vi "Scale Module (Main).vi"(7 "Name of Parent Panel":string="Main.vi", 9 "New Center Coords":T1={"Horizontal"=470, "Vertical"=200}, 10 "Config":variant, 11 "Main UI Message Queue":refnum<queue>) -> ()   [LabVIEW 2018, in "Scale Module.lvlib"]
doc: "This Continuous Measurement sample project is based on the Queued Message Handler template.\n\nThe Event Handling Loop generates messages based on user interface actions.\n\nThe Message Handling Loop processes messages generated by the Event Handling Loop, or by other messages. There are also Acquisition and Logging message handling loop subVIs, and a chart updating loop."
uses:
  Scale Module.lvlib
  support/Message Queue/Message Cluster.ctl
  <vilib>/Utility/miscctls.llb/LVPoint32TypeDef.ctl
  controls/UI State.ctl
  Feed Module/Controls/Scale Module Config Cluster.ctl
  Feed Module/Controls/Scale Module Settings Cluster.ctl
  Mettler Toledo/Controls/Settings Cluster.ctl
  Feed Module/Controls/Scale Module State Cluster.ctl
  Feed Module/Controls/Scale Module Display.ctl
  support/Message Queue/Enqueue Message (Single).vi
  <vilib>/Utility/error.llb/Error Cluster From Error Code.vi
  <vilib>/ErrorRing/Error Ring.xnode
  support/User Event - Stop/User Event - Stop.lvlib
  support/Message Queue/Message Queue.lvlib
  support/Support Library.lvlib
  Measure Instrument/Scale Module Engine.lvlib
  Mettler Toledo/Mettler Toledo.lvlib
  Scale Settings Dialog.vi
  support/Command Log VIs/Command Logging.lvlib
panel:
  in  "Settings Button":bool
  out "ScanCode":i16
  out "g":dbl format="%#_5f"
  out "Log File path":path
  out "Status":string
  in  "Exit":bool
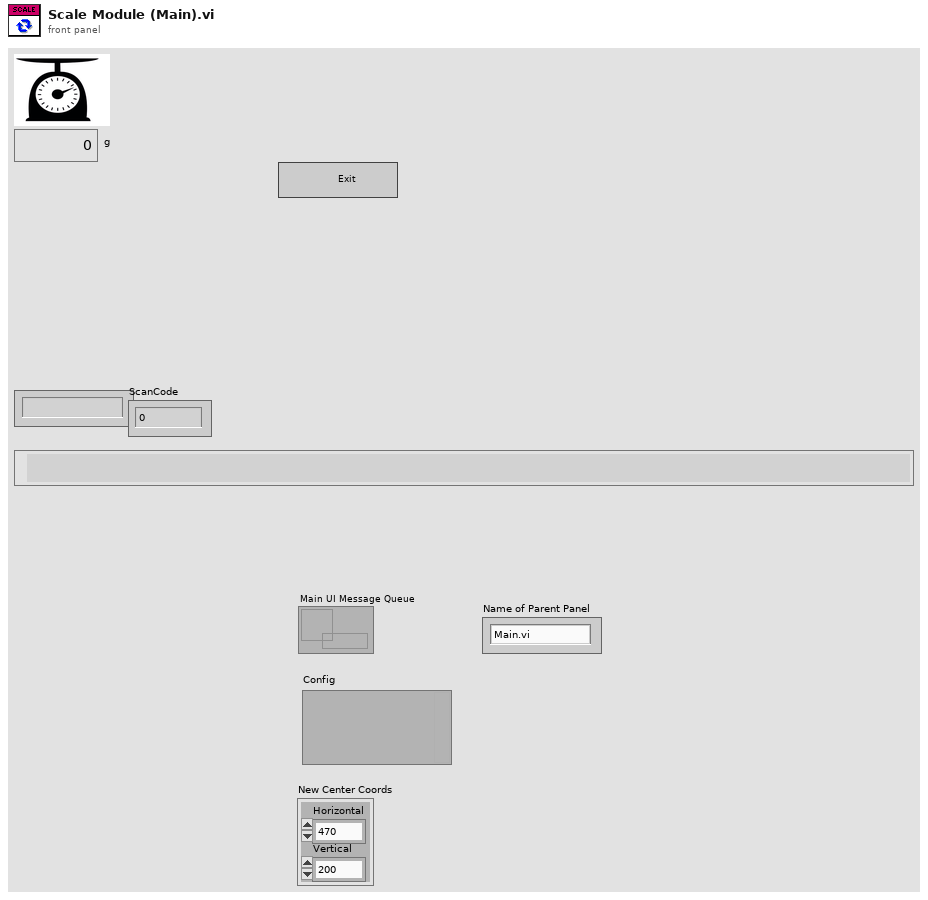
[diagram p1: front panel]
types:
  T1 = typedef "LVPoint32TypeDef.ctl" = cluster{"Horizontal":i32, "Vertical":i32}
  T2 = typedef "Scale Module.lvlib/Scale Module State Cluster.ctl" = cluster{"Scale Module Config":T3}
  T3 = typedef "Scale Module.lvlib/Scale Module Config Cluster.ctl" = cluster{"GUID":string, "Drop Coords":T1, "Process Name":string, "Queue Name":string, "Settings":T4, "Load Count":i32}
  T4 = typedef "Scale Module.lvlib/Scale Module Settings Cluster.ctl" = cluster{"Cycle Period":dbl, "Mettler":T5, "Scale Type":string}
  T5 = typedef "Mettler Toledo.lvlib/Settings Cluster.ctl" = cluster{"VISA resource name":refnum<visa-resource-name>, "Simulated?":bool}
  T6 = typedef "UI State.ctl" = enum16{"Idle", "Acquiring and Logging", "Waiting for Exit", "Waiting for Exit (Acq Stopped)", "Waiting for Exit (Log Stopped)", "Waiting for Stop", "Waiting for Stop (Acq Stopped)", "Waiting for Stop (Log Stopped)"}
  T7 = typedef "Scale Module.lvlib/Scale Message Queues.ctl" = cluster{"Scale UI":refnum<queue>, "Scale Engine":refnum<queue>, "Scale Display":refnum<queue>}
  T8 = typedef "Scale Module.lvlib/Scale Module Display.ctl" = cluster{"Scale Value":dbl, "Cycle Period":dbl}
  T9 = cluster{"Shift":bool, "Ctrl":bool, "Alt":bool, "Cmd":bool, "Opt":bool}
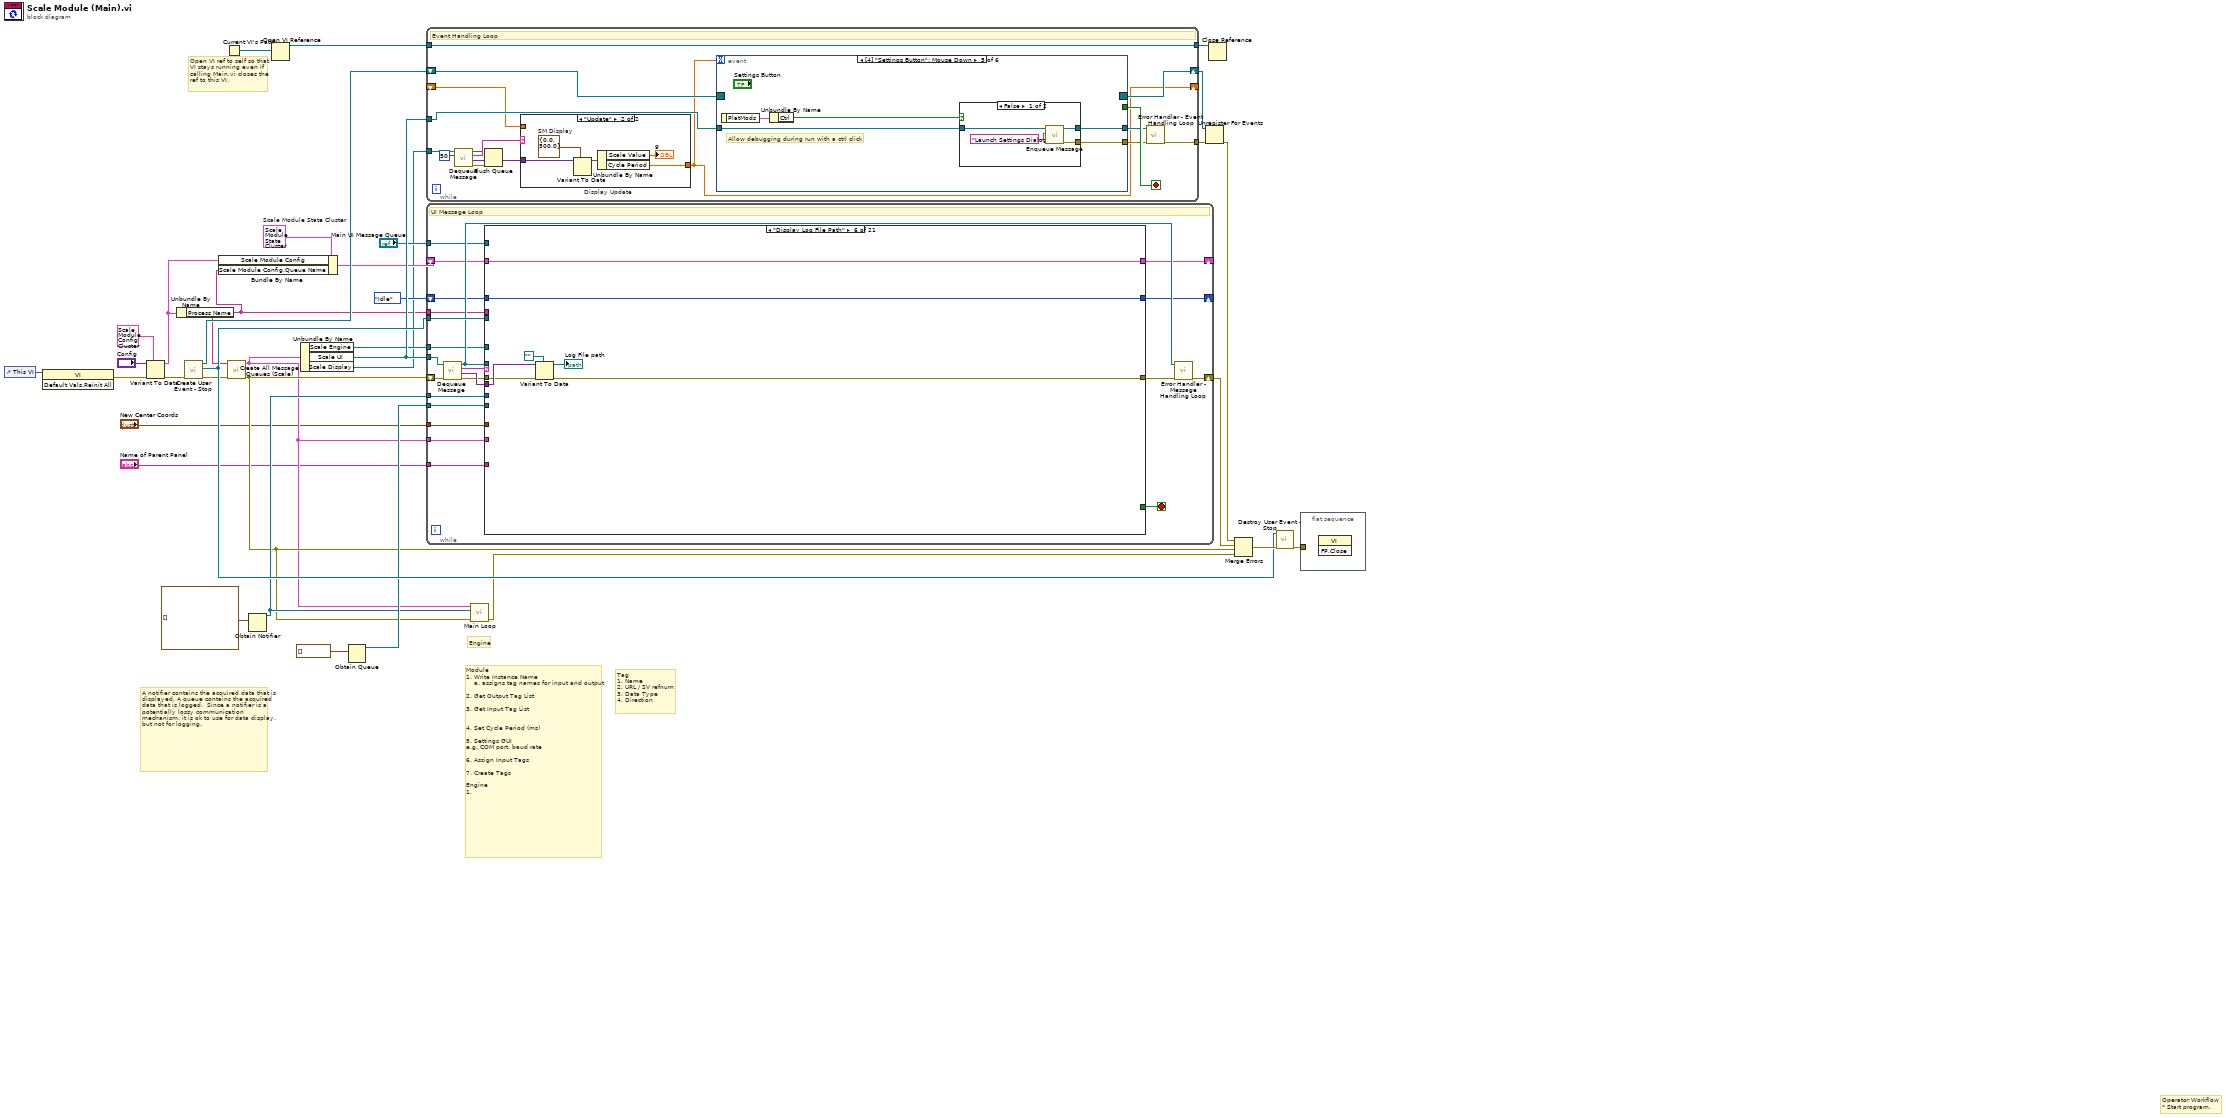
[diagram p0: block diagram]
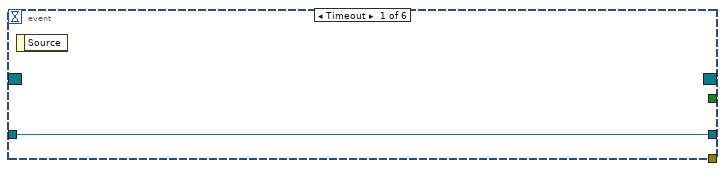
[diagram p3: hidden frame]
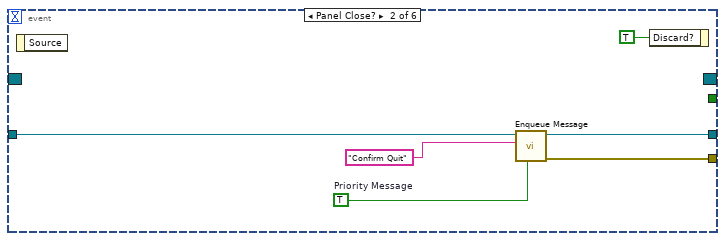
[diagram p4: hidden frame]
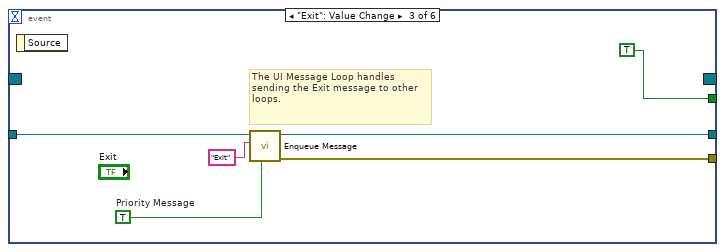
[diagram p5: hidden frame]
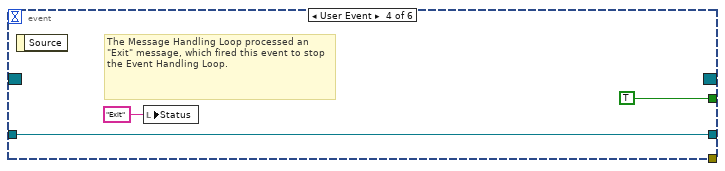
[diagram p6: hidden frame]
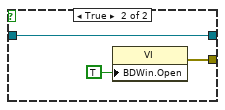
[diagram p7: hidden frame]
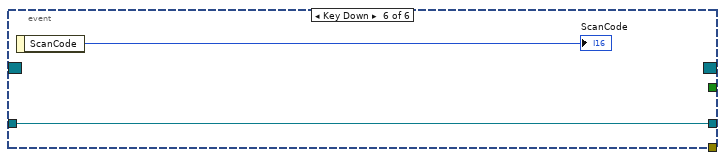
[diagram p8: hidden frame]
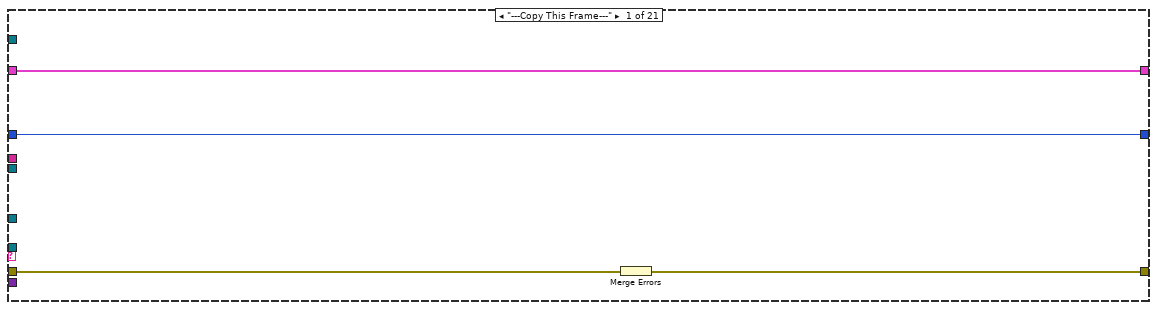
[diagram p9: hidden frame]
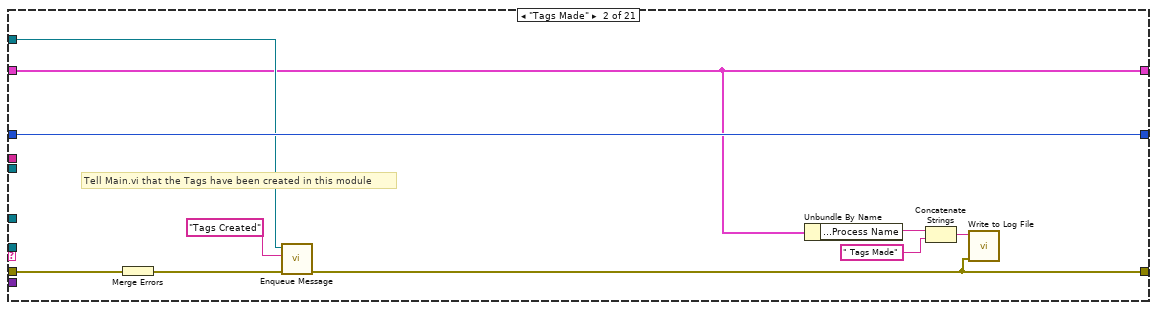
[diagram p10: hidden frame]
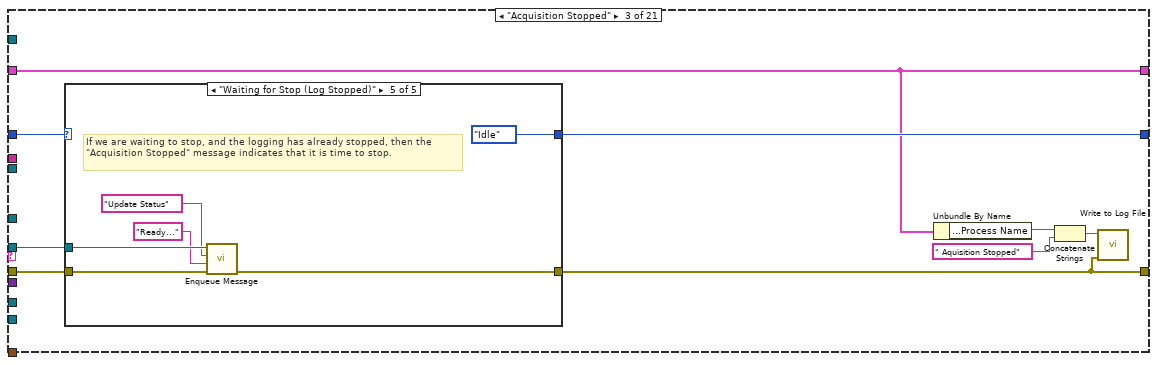
[diagram p11: hidden frame]
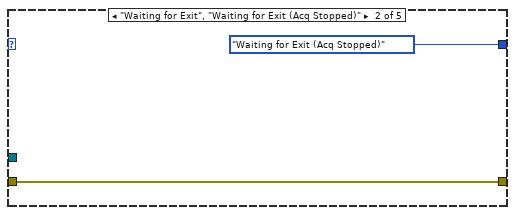
[diagram p13: hidden frame]
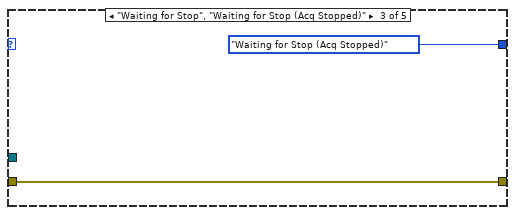
[diagram p14: hidden frame]
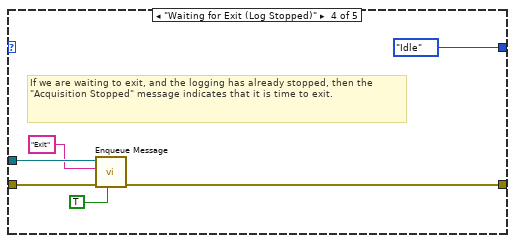
[diagram p15: hidden frame]
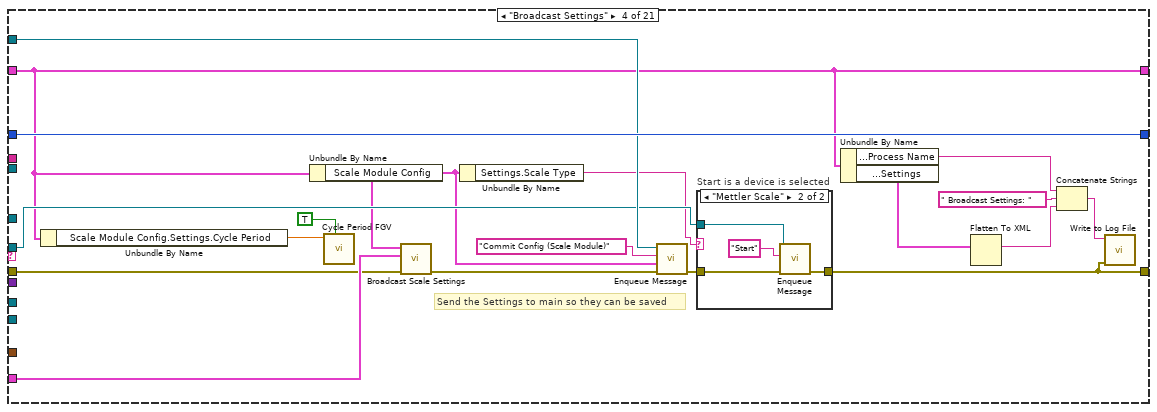
[diagram p16: hidden frame]
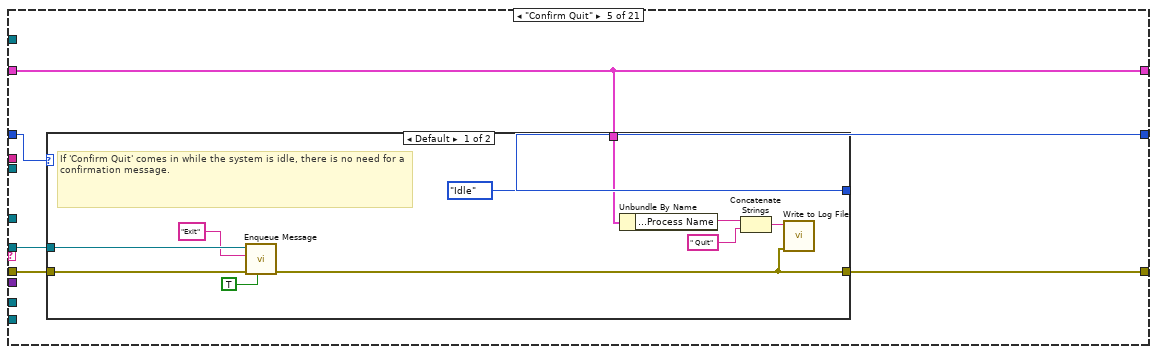
[diagram p18: hidden frame]
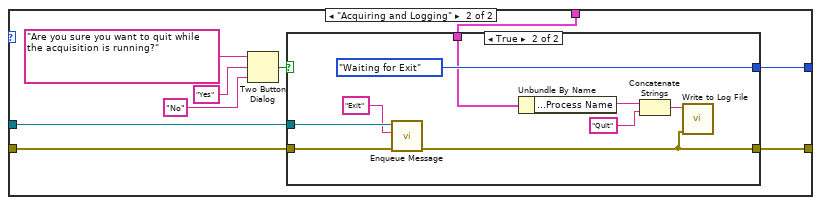
[diagram p19: hidden frame]
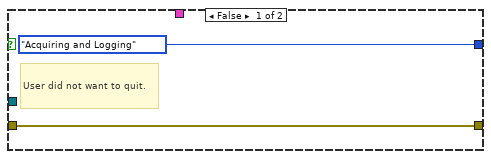
[diagram p20: hidden frame]
diagram:
  w13 = T2 {"Scale Module Config"={"GUID"="PID1-Mettler Toledo Scale 1", "Drop Coords"={"Horizontal"=0, "Vertical"=0}, "Process Name"="PID1-Setpoint", "Queue Name"="", "Settings"={"Cycle Period"=500.0, "Mettler"={"VISA resource name"="", "Simulated?"=FALSE}, "Scale Type"=""}, "Load Count"=0}}  # Scale Module State Cluster
  # "Open VI ref to self so that\nVI stays running even if\ncalling Main.vi closes the\nref to this VI."
  # "Engine"
  # "Operator Workflow\n* Start program."
  # "Module \n1. Write Instance Name\n    a. assigns tag names for input and output\n\n2. Get Output Tag List\n\n3. Get Input Tag List\n\n\n4. Set Cycle Period (ms)\n\n5. Settings GUI\ne.g. COM port, baud rate\n\n6. Assign Input Tags\n\n7. Create Tags\n\nEngine\n1."
  # "Tag\n1. Name\n2. URL / SV refnum\n3. Data Type\n4. Direction"
  # "A notifier contains the acquired data that is displayed. A queue contains the acquired data that is logged.  Since a notifier is a potentially lossy communication mechanism, it is ok to use for data display, but not for logging."
  n1 = control-ref of="This VI"() -> (w10:refnum<vi>)
  n2 = invoke class="VI" method="Default Vals.Reinit All"(reference=w10) -> (error out=w2:errorcluster)  [unwired: 2 in, 2 out]
  n3 = Variant To Data(error in=w2, type=T3 {"GUID"="", "Drop Coords"={"Horizontal"=0, "Vertical"=0}, "Process Name"="", "Queue Name"="", "Settings"={"Cycle Period"=500.0, "Mettler"={"VISA resource name"="", "Simulated?"=FALSE}, "Scale Type"=""}, "Load Count"=0} ("Feed Module Config"), Variant="Config") -> (data=w11:T3, error out=w16:errorcluster)
  n4 = Unbundle By Name(w11) -> ("Process Name"=w1:string)
  n5 = call "Create User Event - Stop.vi"("error in (no error)"=w16) -> ("error out"=w8:errorcluster, "User Event - Stop"=w31:refnum<user-event>, "Stop Event Registration Refnum"=w32:refnum<event-registration>)  [unwired: 8 in]
  n6 = Bundle By Name(cluster=w13, "Scale Module Config"=w11, "Scale Module Config.Queue Name"=w1) -> (w17:T2)
  n7 = Current VI's Path() -> (path=w18:path)
  n8 = call "Create All Message Queues (Scale).vi"("error in (no error)"=w8, "Process Name"=w1) -> ("error out"=w7:errorcluster, "Message Queues"=w6:T7)  [unwired: 8 in]
  n9 = Obtain Notifier(notification data type=waveform(dbl)[] []) -> (notifier out=w21:refnum<notifier>)  [unwired: 3 in, 2 out]
  n10 = Open VI Reference(vi path=w18) -> (vi reference=w19:refnum<vi>)  [unwired: 5 in, 1 out]
  n11 = Unbundle By Name(w6) -> ("Scale Engine"=w24:refnum<queue>, "Scale UI"=w28:refnum<queue>, "Scale Display"=w12:refnum<queue>)
  n12 = Obtain Queue(element data type=waveform(dbl)[] []) -> (queue out=w23:refnum<queue>)  [unwired: 4 in, 2 out]
  n13 = while {
    tunnel: w28 -> [w52]
    tunnel: w31 -> [w56]
    shift-right: [w48] -> w35
    shift-left: w7 -> [w55]
    shift-right: [w39] -> _
    shift-left: w17 -> [w41]
    tunnel: w21 -> [w51]
    tunnel: w23 -> [w50]
    shift-right: [w45] -> _
    shift-left: UI_State."Idle" ("UI State") -> [w46]
    tunnel: w24 -> [w44]
    tunnel: w6 -> [w43]
    tunnel: "Main UI Message Queue" -> [w40]
    tunnel: w1 -> [w38]
    tunnel: "New Center Coords" -> [w37]
    tunnel: "Name of Parent Panel" -> [w36]
    stop <- w57 stop-if-true
    # "UI Message Loop"
    n14 = call "Dequeue Message.vi"("error in (no error)"=w55, "Message Queue"=w52) -> ("error out"=w42:errorcluster, "Message Data"=w53:variant, "Message"=w54:string, "dup Message Queue"=w47:refnum<queue>)  [unwired: 6 in]
    n15 = case "Message Cases" shown="\"Display Log File Path\"" w54 {
      selector: w54 -> [_ _ _ _ _ _ _ _ _ _ _ _ _ _ _ _ _ _ _ _ w393]
      tunnel: w47 -> [_ _ w77 w109 w127 _ w177 w191 w213 _ w252 w269 w286 w309 w317 w335 _ _ w382 _ _]
      tunnel: w42 -> [w61 w71 w78 w113 w126 w161 w172 w195 w212 w238 w248 w267 w287 w310 w316 w334 w341 w358 w377 w391 _]
      tunnel: [w60 w62 w73 w102 w125 w162 w167 w182 w197 w238 w240 w260 w282 w308 w315 w330 w346 w353 w369 w392 w395] -> w49
      tunnel: [_ _ _ _ _ _ _ _ TRUE _ _ _ _ _ _ _ _ _ _ _ _] -> w57
      tunnel: w53 -> [_ _ _ _ _ w164 _ w194 w202 _ _ _ _ _ _ _ _ _ _ w390 _]
      tunnel: w56 -> [_ _ _ _ _ _ _ _ w223 _ _ _ _ _ _ _ _ _ _ _ _]
      tunnel: w41 -> [w58 w63 w72 w101 w123 w159 w166 w181 w196 w235 w239 w271 w281 w314 w321 w329 w339 w352 w368 w385 w394]
      tunnel: w51 -> [_ _ _ _ _ _ _ _ w221 _ _ _ _ _ _ _ _ _ _ _ _]
      tunnel: w50 -> [_ _ _ _ _ _ _ _ w217 _ _ _ _ _ _ _ _ _ _ _ _]
      tunnel: w46 -> [w59 w70 w80 w117 w128 w160 w173 w186 w210 _ _ w275 w289 w313 w320 _ _ _ w378 w386 w399]
      tunnel: [w59 w70 w79 w117 w124 w160 w174 w186 w209 UI_State."Idle" ("UI State") UI_State."Idle" ("UI State") w275 w288 w313 w320 UI_State."Acquiring and Logging" ("UI State") UI_State."Acquiring and Logging" ("UI State") UI_State."Acquiring and Logging" ("UI State") w379 w386 w399] -> w45
      tunnel: w44 -> [_ _ _ _ _ _ _ _ w216 _ _ _ _ _ _ _ w344 w361 w376 _ _]
      tunnel: w43 -> [_ _ _ w116 _ _ _ _ _ _ _ _ _ _ _ _ _ _ _ _ _]
      tunnel: w40 -> [_ w67 _ w110 _ _ _ _ w201 _ _ w272 _ _ _ _ _ _ _ _ _]
      tunnel: [w58 w63 w72 w101 w123 w159 w166 w181 w196 w235 w239 w259 w281 w314 w321 w329 w339 w352 w368 w385 w394] -> w39
      tunnel: w38 -> [_ _ _ _ _ _ _ _ _ _ w246 _ _ _ _ _ _ _ _ _ _]
      tunnel: w37 -> [_ _ _ _ _ _ _ _ _ _ w245 _ _ _ _ _ _ _ _ _ _]
      tunnel: w36 -> [_ _ _ _ _ _ _ _ _ _ w244 _ _ _ _ _ _ _ _ _ _]
      frame "---Copy This Frame---" {
        # "Duplicate this frame when creating new messages.  Change this comment in the duplicated frame to describe this message."
        n16 = Merge Errors(w61) -> (w60:errorcluster)
      }
      frame "Tags Made" {
        # "Tell Main.vi that the Tags have been created in this module"
        # "Duplicate this frame when creating new messages.  Change this comment in the duplicated frame to describe this message."
        n17 = Merge Errors(w71) -> (w68:errorcluster)
        n18 = call-poly "Enqueue Message.vi"("error in (no error)"=w68, "Message"="Tags Created", "Message Queue"=w67) -> ("error out"=w62:errorcluster)  [unwired: 7 in, 1 out]
        n19 = Unbundle By Name(w63) -> ("Scale Module Config.Process Name"=w66:string)
        n20 = Concatenate Strings(w66, " Tags Made" ("text")) -> (w64:string)
        n21 = call "Write to Log File.vi"("error in"=w62, "text"=w64) -> ()  [unwired: 9 in, 1 out]
      }
      frame "Acquisition Stopped" {
        # "Logic for determining what action to take when the acquisition has stopped."
        n22 = case shown="\"Waiting for Stop (Log Stopped)\"" w80 {
          selector: w80 -> [w82 _ _ _ _]
          tunnel: [w82 UI_State."Waiting for Exit (Acq Stopped)" ("UI State") UI_State."Waiting for Stop (Acq Stopped)" ("UI State") UI_State."Idle" ("UI State") UI_State."Idle" ("UI State")] -> w79
          tunnel: w78 -> [w81 w83 w85 w91 w97]
          tunnel: [w81 w83 w85 w90 w96] -> w73
          tunnel: w77 -> [_ _ _ w89 w95]
          frame Default {
          }
          frame "Waiting for Exit", "Waiting for Exit (Acq Stopped)" {
          }
          frame "Waiting for Stop", "Waiting for Stop (Acq Stopped)" {
          }
          frame "Waiting for Exit (Log Stopped)" {
            # "If we are waiting to exit, and the logging has already stopped, then the \"Acquisition Stopped\" message indicates that it is time to exit."
            n23 = call-poly "Enqueue Message.vi"("Priority Message? (F)"=TRUE, "error in (no error)"=w91, "Message"="Exit", "Message Queue"=w89) -> ("error out"=w90:errorcluster)  [unwired: 6 in, 1 out]
          }
          frame "Waiting for Stop (Log Stopped)" {
            # "If we are waiting to stop, and the logging has already stopped, then the \"Acquisition Stopped\" message indicates that it is time to stop."
            n24 = call-poly "Enqueue Message.vi"("error in (no error)"=w97, "Message Data"="Ready..." ("Message"), "Message"="Update Status", "Message Queue"=w95) -> ("error out"=w96:errorcluster)  [unwired: 6 in, 1 out]
          }
        }
        n25 = Unbundle By Name(w72) -> ("Scale Module Config.Process Name"=w76:string)
        n26 = Concatenate Strings(w76, " Aquisition Stopped" ("text")) -> (w74:string)
        n27 = call "Write to Log File.vi"("error in"=w73, "text"=w74) -> ()  [unwired: 9 in, 1 out]
      }
      frame "Broadcast Settings" {
        # "Send the Settings to main so they can be saved"
        # "Send the 'Update Settings' message to the Logging and Acquisition message loops."
        n28 = Unbundle By Name(w101) -> ("Scale Module Config.Settings.Cycle Period"=w114:dbl)
        n29 = Unbundle By Name(w101) -> ("Scale Module Config"=w106:T3)
        n30 = call "Cycle Period FGV.vi"("Write"=TRUE, "Cycle Period In (ms)"=w114) -> ()  [unwired: 8 in, 2 out]
        n31 = call "Broadcast Scale Settings.vi"("error in (no error)"=w113, "Message Queues"=w116, "Scale Module Config"=w106) -> ("error out"=w111:errorcluster)  [unwired: 8 in]
        n32 = Unbundle By Name(w106) -> ("Settings.Scale Type"=w107:string)
        n33 = call-poly "Enqueue Message.vi"("error in (no error)"=w111, "Message Data"=w106, "Message"="Commit Config (Scale Module)", "Message Queue"=w110) -> ("error out"=w108:errorcluster)  [unwired: 6 in, 1 out]
        n34 = case "Start is a device is selected" shown="\"Mettler Scale\"" w107 {
          tunnel: w109 -> [_ w121]
          tunnel: w108 -> [w118 w120]
          tunnel: [w118 w119] -> w102
          frame "False", Default {
          }
          frame "Mettler Scale" {
            n35 = call-poly "Enqueue Message.vi"("error in (no error)"=w120, "Message"="Start", "Message Queue"=w121) -> ("error out"=w119:errorcluster)  [unwired: 7 in, 1 out]
          }
        }
        n36 = Unbundle By Name(w101) -> ("Scale Module Config.Process Name"=w105:string, "Scale Module Config.Settings"=w100:T4)
        n37 = Flatten To XML(anything=w100) -> (xml string=w99:string)
        n38 = Concatenate Strings(w105, " Broadcast Settings: " ("text"), w99) -> (w103:string)
        n39 = call "Write to Log File.vi"("error in"=w102, "text"=w103) -> ()  [unwired: 9 in, 1 out]
      }
      frame "Confirm Quit" {
        # "Confirm Quit - Message that can confirm whether or not the user wants to exit the application."
        n40 = case shown="Default" w128 {
          tunnel: w127 -> [w137 w144]
          tunnel: w126 -> [w136 w142]
          tunnel: [w130 w141] -> w125
          tunnel: [UI_State."Idle" ("UI State") w140] -> w124
          tunnel: w123 -> [w129 w139]
          frame Default {
            # "If 'Confirm Quit' comes in while the system is idle, there is no need for a confirmation message."
            n41 = call-poly "Enqueue Message.vi"("Priority Message? (F)"=TRUE, "error in (no error)"=w136, "Message"="Exit", "Message Queue"=w137) -> ("error out"=w130:errorcluster)  [unwired: 6 in, 1 out]
            n42 = Unbundle By Name(w129) -> ("Scale Module Config.Process Name"=w133:string)
            n43 = Concatenate Strings(w133, " Quit" ("text")) -> (w131:string)
            n44 = call "Write to Log File.vi"("error in"=w130, "text"=w131) -> ()  [unwired: 9 in, 1 out]
          }
          frame "Acquiring and Logging" {
            n45 = Two Button Dialog(message="Are you sure you want to quit while the acquisition is running?" ("Confirm Quit Message"), 1:"No" ("No"), 2:"Yes" ("Yes")) -> (T button?=w143:bool)
            n46 = case shown="True" w143 {
              tunnel: w144 -> [_ w158]
              tunnel: w142 -> [w148 w157]
              tunnel: [w148 w151] -> w141
              tunnel: [UI_State."Acquiring and Logging" ("UI State") UI_State."Waiting for Exit" ("UI State")] -> w140
              tunnel: w139 -> [_ w150]
              frame False {
                # "User did not want to quit."
              }
              frame True {
                n47 = call-poly "Enqueue Message.vi"("error in (no error)"=w157, "Message"="Exit", "Message Queue"=w158) -> ("error out"=w151:errorcluster)  [unwired: 7 in, 1 out]
                n48 = Unbundle By Name(w150) -> ("Scale Module Config.Process Name"=w154:string)
                n49 = Concatenate Strings(w154, "Quit" ("text")) -> (w152:string)
                n50 = call "Write to Log File.vi"("error in"=w151, "text"=w152) -> ()  [unwired: 9 in, 1 out]
              }
            }
          }
        }
      }
      frame "Display Log File Path" {
        n51 = Variant To Data(error in=w161, type=path "", Variant=w164) -> (data=→"Log File path":path, error out=w162:errorcluster)
      }
      frame "E-Stop" {
        # "E-Stop has no effect on the scale"
        # "Message Acquisition and Logging loops to stop"
        # "Stop the pumps."
        n52 = call-poly "Enqueue Message.vi"("error in (no error)"=w172, "Message Data"="Ready..." ("Ready..."), "Message"="Update Status", "Message Queue"=w177) -> ("error out"=w171:errorcluster)  [unwired: 6 in, 1 out]
        n53 = case shown="\"Waiting for Exit\"" w173 {
          selector: w173 -> [_ w179]
          tunnel: [UI_State."Waiting for Stop" ("UI State") w179] -> w174
          frame Default {
          }
          frame "Waiting for Exit" {
          }
        }
        n54 = Merge Errors(w171) -> (w167:errorcluster)
        n55 = Unbundle By Name(w166) -> ("Scale Module Config.Process Name"=w170:string)
        n56 = Concatenate Strings(w170, " E-STOP" ("text")) -> (w168:string)
        n57 = call "Write to Log File.vi"("error in"=w167, "text"=w168) -> ()  [unwired: 9 in, 1 out]
      }
      frame "Error" {
        # "Error - Check the error message data and respond accordingly. This message is sent by the \"Error Handler\" VIs at the end of each loop in this application."
        n58 = Variant To Data(error in=w195, type=errorcluster {"status"=FALSE, "code"=0, "source"=""} ("error out"), Variant=w194) -> (data=w192:errorcluster, error out=w188:errorcluster)
        n59 = call <vilib>:"General Error Handler.vi"("error in (no error)"=w192) -> ("message"=w180:string)  [unwired: 10 in, 4 out]
        n60 = call-poly "Enqueue Message.vi"("Priority Message? (F)"=TRUE, "Message"="Exit", "Message Queue"=w191) -> ("error out"=w187:errorcluster)  [unwired: 7 in, 1 out]
        n61 = Merge Errors(w187, w188) -> (w182:errorcluster)
        n62 = Unbundle By Name(w181) -> ("Scale Module Config.Process Name"=w185:string)
        n63 = Concatenate Strings(w185, " Error: " ("text"), w180) -> (w183:string)
        n64 = call "Write to Log File.vi"("error in"=w182, "text"=w183) -> ()  [unwired: 9 in, 1 out]
      }
      frame "Exit" {
        w205 = TRUE  # Delete Module?
        # "Don't check the error outs. The acquisition and logging queues may have already been released."
        # "Close references owned by the Main VI."
        # "Stop the VI"
        # "Exit - Fire the User Event to stop the Event Handling Loop.  Also send Exit messages to the Acquisition and Logging loops."
        n65 = call "Fire User Event - Stop.vi"("User Event - Stop"=w223) -> ("error out"=w222:errorcluster)  [unwired: 10 in]
        n66 = Build Array(w216) -> (w215:refnum<queue>[])
        n67 = for {
          tunnel: w215 -> [w232] mode=indexing
          n68 = call-poly "Enqueue Message.vi"("Message"="Stop", "Message Queue"=w232) -> ("dup Message Queue"=w233:refnum<queue>)  [unwired: 8 in, 1 out]
          n69 = call-poly "Enqueue Message.vi"("Message"="Exit", "Message Queue"=w233) -> ()  [unwired: 8 in, 2 out]
        }
        n70 = Variant To Data(type=w205, Variant=w202) -> (data=w204:bool, error out=w206:errorcluster)  [unwired: 1 in]
        n71 = call-poly "Enqueue Message.vi"("error in (no error)"=w212, "Message Data"="Ready..." ("Ready..."), "Message"="Update Status", "Message Queue"=w213) -> ("error out"=w211:errorcluster, "dup Message Queue"=w208:refnum<queue>)  [unwired: 6 in]
        n72 = Select(t=w205, s=w206, f=w204) -> (s? t:f=w203:bool)
        n73 = case "Don't enqueue Delete Module if opening campaign because it\nwill already have been deleted and new config loaded and we create\na race condition." shown="True" w203 {
          tunnel: w201 -> [_ w227]
          tunnel: w196 -> [_ w226]
          frame False {
          }
          frame True {
            n74 = Unbundle By Name(w226) -> ("Scale Module Config.GUID"=w225:string)
            n75 = call-poly "Enqueue Message.vi"("Message Data"=w225, "Message"="Delete Module", "Message Queue"=w227) -> ()  [unwired: 7 in, 2 out]
          }
        }
        n76 = Release Queue(queue=w208, error in (no error)=w211) -> (error out=w220:errorcluster)  [unwired: 1 in, 2 out]
        n77 = Release Notifier(notifier=w221, error in (no error)=w220) -> (error out=w219:errorcluster)  [unwired: 1 in, 2 out]
        n78 = Release Queue(queue=w217, error in (no error)=w219) -> (error out=w218:errorcluster)  [unwired: 1 in, 2 out]
        n79 = Merge Errors(w222, w218) -> (w197:errorcluster)
        n80 = case shown="Default" w210 {
          selector: w210 -> [_ w230]
          tunnel: [UI_State."Waiting for Stop" ("UI State") w230] -> w209
          frame Default {
          }
          frame "Waiting for Exit" {
          }
        }
        n81 = Unbundle By Name(w196) -> ("Scale Module Config.Process Name"=w200:string)
        n82 = Concatenate Strings(w200, " Exit" ("text")) -> (w198:string)
        n83 = call "Write to Log File.vi"("error in"=w197, "text"=w198) -> ()  [unwired: 9 in, 1 out]
      }
      frame "Init UI Refs" {
        # "Init UI Refs - Store control references for UI controls.  Also enable/disable controls appropriately."
        n84 = property class="VI"("Front Panel.Closeable"=TRUE ("Front Panel Window:Closeable")) -> ()  [unwired: 2 in, 2 out]
      }
      frame "Initialize" {
        # "Initialize - Get configuration settings, then message the UI to initialize, and broadcast the settings to the other message loops."
        n85 = call-poly "Enqueue Message.vi"("error in (no error)"=w248, "Message"="Init UI Refs", "Message Queue"=w252) -> ("error out"=w250:errorcluster, "dup Message Queue"=w251:refnum<queue>)  [unwired: 7 in]
        n86 = property class="VI" props=["FP.State"]() -> (reference out=w247:refnum<vi>)  [unwired: 2 in, 2 out]
        n87 = call "Make Child and Move.vi"("Process Name"=w246, "Name of Parent Panel"=w244, "New Center Coords"=w245, "VI in"=w247) -> ()  [unwired: 8 in]
        n88 = call-poly "Enqueue Message.vi"("error in (no error)"=w250, "Message"="Broadcast Settings", "Message Queue"=w251) -> ("error out"=w258:errorcluster, "dup Message Queue"=w257:refnum<queue>)  [unwired: 7 in]
        n89 = call-poly "Enqueue Message.vi"("error in (no error)"=w258, "Message Data"="Ready..." ("Ready..."), "Message"="Update Status", "Message Queue"=w257) -> ("error out"=w240:errorcluster)  [unwired: 6 in, 1 out]
        n90 = Unbundle By Name(w239) -> ("Scale Module Config.Process Name"=w243:string)
        n91 = Concatenate Strings(w243, " Initialize" ("text")) -> (w241:string)
        n92 = call "Write to Log File.vi"("error in"=w240, "text"=w241) -> ()  [unwired: 9 in, 1 out]
      }
      frame "Launch Settings Dialog" {
        # "Launch the Settings Dialog when the user clicks the 'Settings' button."
        n93 = Unbundle By Name(w271) -> ("Scale Module Config"=w270:T3)
        n94 = Unbundle By Name(w270) -> ("Load Count"=w273:i32)
        n95 = Increment(x=w273) -> (x+1=w274:i32)
        n96 = Bundle By Name(cluster=w270, "Load Count"=w274) -> (w268:T3)
        n97 = call-by-ref "?"("error in (no error)"=w267, "Scale Module Config In"=w268) -> ("error out"=w266:errorcluster, "Cancelled?"=w264:bool, "Scale Module Config Out"=w265:T3)  [unwired: 8 in, 3 out]
        n98 = case shown="False" w264 {
          tunnel: w266 -> [w277 w280]
          tunnel: [w276 w280] -> w260
          tunnel: w272 -> [_ _]
          tunnel: w269 -> [w279 _]
          tunnel: w265 -> [_ _]
          frame False {
            n99 = call-poly "Enqueue Message.vi"("error in (no error)"=w277, "Message"="Broadcast Settings", "Message Queue"=w279) -> ("error out"=w276:errorcluster)  [unwired: 7 in, 1 out]
          }
          frame True {
          }
        }
        n100 = Bundle By Name(cluster=w271, "Scale Module Config"=w265) -> (w259:T2)
        n101 = Unbundle By Name(w259) -> ("Scale Module Config.Process Name"=w263:string)
        n102 = Concatenate Strings(w263, " Setting Dialog Launched" ("text")) -> (w261:string)
        n103 = call "Write to Log File.vi"("error in"=w260, "text"=w261) -> ()  [unwired: 9 in, 1 out]
      }
      frame "Logging Stopped" {
        # "Logic for determining what action to take when the logging has stopped."
        n104 = case shown="\"Waiting for Exit (Acq Stopped)\"" w289 {
          selector: w289 -> [w291 _ _ _ _]
          tunnel: [w291 UI_State."Waiting for Exit (Log Stopped)" ("UI State") UI_State."Waiting for Stop (Log Stopped)" ("UI State") UI_State."Idle" ("UI State") UI_State."Idle" ("UI State")] -> w288
          tunnel: w287 -> [w290 w292 w294 w300 w306]
          tunnel: [w290 w292 w294 w299 w305] -> w282
          tunnel: w286 -> [_ _ _ w298 w304]
          frame Default {
          }
          frame "Waiting for Exit", "Waiting for Exit (Log Stopped)" {
          }
          frame "Waiting for Stop", "Waiting for Stop (Log Stopped)" {
          }
          frame "Waiting for Exit (Acq Stopped)" {
            # "If we are waiting to exit, and the acquisition has already stopped, then the \"Logging Stopped\" message indicates that it is time to exit."
            n105 = call-poly "Enqueue Message.vi"("Priority Message? (F)"=TRUE, "error in (no error)"=w300, "Message"="Exit", "Message Queue"=w298) -> ("error out"=w299:errorcluster)  [unwired: 6 in, 1 out]
          }
          frame "Waiting for Stop (Acq Stopped)" {
            # "If we are waiting to stop, and the acquisition has already stopped, then the \"Logging Stopped\" message indicates that it is time to stop."
            n106 = call-poly "Enqueue Message.vi"("error in (no error)"=w306, "Message Data"="Ready..." ("Message"), "Message"="Update Status", "Message Queue"=w304) -> ("error out"=w305:errorcluster)  [unwired: 6 in, 1 out]
          }
        }
        n107 = Unbundle By Name(w281) -> ("Scale Module Config.Process Name"=w285:string)
        n108 = Concatenate Strings(w285, " Logging Stopped" ("text")) -> (w283:string)
        n109 = call "Write to Log File.vi"("error in"=w282, "text"=w283) -> ()  [unwired: 9 in, 1 out]
      }
      frame "Send to Sequencer" {
        n110 = local read "g"() -> (w311:dbl)
        n111 = call-poly "Enqueue Message.vi"("error in (no error)"=w310, "Message Data"=w311, "Message"="Sent to Sequence", "Message Queue"=w309) -> ("error out"=w308:errorcluster)  [unwired: 6 in, 1 out]
      }
      frame "Sent to Sequence" {
        n112 = local read "g"() -> (w318:dbl)
        n113 = flat-sequence {
          tunnel: w316 -> [w326]
          tunnel: w317 -> [w324]
          tunnel: [w325] -> w319
          tunnel: w318 -> [w322]
          tunnel: [w328] -> w315
          tunnel: w319 -> [w328]
          frame #0 {
            n114 = call-poly "Enqueue Message.vi"("error in (no error)"=w326, "Message Data"=w322, "Message"="Sent to Sequence", "Message Queue"=w324) -> ("error out"=w325:errorcluster)  [unwired: 6 in, 1 out]
          }
          frame #1 {
            n115 = Wait (ms)(milliseconds to wait=u32 50) -> ()  [unwired: 1 out]
          }
        }
      }
      frame "Start" {
        # "Message Acquisition and Logging loops to start"
        # "Start - Enable/Disable buttons appropriately for an acquisition that has started, and update status display."
        n116 = call-poly "Enqueue Message.vi"("error in (no error)"=w334, "Message"="Start Loops", "Message Queue"=w335) -> ("error out"=w336:errorcluster)  [unwired: 7 in, 1 out]
        n117 = Merge Errors(w336) -> (w330:errorcluster)
        n118 = Unbundle By Name(w329) -> ("Scale Module Config.Process Name"=w333:string)
        n119 = Concatenate Strings(w333, " Start" ("text")) -> (w331:string)
        n120 = call "Write to Log File.vi"("error in"=w330, "text"=w331) -> ()  [unwired: 9 in, 1 out]
      }
      frame "Start Loops" {
        # "I'm not sure what we would have multiple Process names in a module for but i'll leave it for now."
        # "Message Acquisition and Logging loops to start"
        # "Start - Enable/Disable buttons appropriately for an acquisition that has started, and update status display."
        n121 = Unbundle By Name(w339) -> ("Scale Module Config.Process Name"=w340:string)
        n122 = Build Array(w344) -> (w342:refnum<queue>[])
        n123 = property class="VI"("Front Panel.Title"=w340) -> ()  [unwired: 2 in, 2 out]
        n124 = for {
          tunnel: w341 -> [w350]
          tunnel: [w349] -> w343 mode=indexing
          tunnel: w342 -> [w348] mode=indexing
          tunnel: w340 -> [w347]
          n125 = call-poly "Enqueue Message.vi"("error in (no error)"=w350, "Message Data"=w347, "Message"="Start", "Message Queue"=w348) -> ("error out"=w349:errorcluster)  [unwired: 6 in, 1 out]
        }
        n126 = Merge Errors(w343) -> (w346:errorcluster)
      }
      frame "Start Log" {
        # "I'm not sure what we would have multiple Process names in a module for but i'll leave it for now."
        # "Message Acquisition and Logging loops to start"
        # "Start - Enable/Disable buttons appropriately for an acquisition that has started, and update status display."
        n127 = Unbundle By Name(w352) -> ("Scale Module Config.Process Name"=w357:string)
        n128 = Build Array(w361) -> (w359:refnum<queue>[])
        n129 = property class="VI"("Front Panel.Title"=w357) -> ()  [unwired: 2 in, 2 out]
        n130 = for {
          tunnel: w358 -> [w366]
          tunnel: [w365] -> w360 mode=indexing
          tunnel: w359 -> [w364] mode=indexing
          tunnel: w357 -> [w363]
          n131 = call-poly "Enqueue Message.vi"("error in (no error)"=w366, "Message Data"=w363, "Message"="Start Log", "Message Queue"=w364) -> ("error out"=w365:errorcluster)  [unwired: 6 in, 1 out]
        }
        n132 = Merge Errors(w360) -> (w353:errorcluster)
        n133 = Unbundle By Name(w352) -> ("Scale Module Config.Process Name"=w356:string)
        n134 = Concatenate Strings(w356, " Start Log" ("text")) -> (w354:string)
        n135 = call "Write to Log File.vi"("error in"=w353, "text"=w354) -> ()  [unwired: 9 in, 1 out]
      }
      frame "Stop" {
        # "Stop - Enable/Disable buttons appropriately for an acquisition that has stopped, and update status display."
        n136 = call-poly "Enqueue Message.vi"("error in (no error)"=w377, "Message Data"="Ready..." ("Ready..."), "Message"="Update Status", "Message Queue"=w382) -> ("error out"=w375:errorcluster)  [unwired: 6 in, 1 out]
        n137 = call-poly "Enqueue Message.vi"("error in (no error)"=w375, "Message"="Stop", "Message Queue"=w376) -> ("error out"=w373:errorcluster)  [unwired: 7 in, 1 out]
        n138 = case shown="Default" w378 {
          selector: w378 -> [_ w384]
          tunnel: [UI_State."Waiting for Stop" ("UI State") w384] -> w379
          frame Default {
          }
          frame "Waiting for Exit" {
          }
        }
        n139 = Merge Errors(w373) -> (w369:errorcluster)
        n140 = Unbundle By Name(w368) -> ("Scale Module Config.Process Name"=w372:string)
        n141 = Concatenate Strings(w372, " Stop" ("text")) -> (w370:string)
        n142 = call "Write to Log File.vi"("error in"=w369, "text"=w370) -> ()  [unwired: 9 in, 1 out]
      }
      frame "Update Status" {
        # "Update Display - Convert the message data to a string to display in the Status indicator."
        n143 = Variant To Data(error in=w391, type="", Variant=w390) -> (data=→"Status":string, error out=w388:errorcluster)
        n144 = Merge Errors(w388) -> (w392:errorcluster)
      }
      frame Default {
        # "'Default' case only runs if there is a message that isn't defined in any of the other cases.  Output a programming error."
        n145 = xnode "Error Ring"("parameter 0"=w393) -> ("error out"=w395:errorcluster)
        n146 = Unbundle By Name(w394) -> ("Scale Module Config.Process Name"=w398:string)
        n147 = Concatenate Strings(w398, "Invalid Message Recieved" ("text"), w393) -> (w396:string)
        n148 = call "Write to Log File.vi"("error in"=w395, "text"=w396) -> ()  [unwired: 9 in, 1 out]
      }
    }
    n149 = call "Error Handler - Message Handling Loop.vi"("error in (no error)"=w49, "Message Queue"=w47) -> ("dup error in"=w48:errorcluster)  [unwired: 8 in, 1 out]
  }
  n150 = while {
    tunnel: w28 -> [w416]
    tunnel: [w418] -> w34
    shift-right: [w417] -> w29
    shift-left: w32 -> [w422]
    tunnel: [w415] -> w20
    tunnel: w19 -> [w415]
    tunnel: w12 -> [w414]
    shift-right: [w411] -> _
    shift-left: _ -> [w410]
    stop <- w421 stop-if-true
    # "Event Handling Loop"
    n151 = call "Dequeue Message.vi"("timeout in ms (-1)"=50, "Message Queue"=w414) -> ("error out"=w407:errorcluster, "Message Data"=w412:variant, "Message"=w413:string, "dup Message Queue"=w408:refnum<queue>)  [unwired: 6 in]
    n152 = Flush Queue(queue=w408, error in (no error)=w407) -> ()  [unwired: 3 out]
    n153 = case "Display Update" shown="\"Update\"" w413 {
      tunnel: w412 -> [_ w428]
      tunnel: [w423 w425] -> w411
      tunnel: w410 -> [w423 _]
      frame "False", Default {
      }
      frame "Update" {
        w424 = T8 {"Scale Value"=0.0, "Cycle Period"=500.0}  # SM Display
        n154 = Variant To Data(type=w424, Variant=w428) -> (data=w427:T8)  [unwired: 1 in, 1 out]
        n155 = Unbundle By Name(w427) -> ("Scale Value"=→"g":dbl, "Cycle Period"=w425:dbl)
      }
    }
    n156 = event shown="[4] \"Settings Button\": Mouse Down" {
      selector: w422 -> [_ _ _ _ _ _]
      dyn-events: [_ _ _ _ _ _] -> w417
      timeout: w411 -> [_ _ _ _ _ _]
      tunnel: [_ _ TRUE ("Discard?") TRUE ("Discard?") _ _] -> w421
      tunnel: w416 -> [w429 w432 w436 w442 w447 w457]
      tunnel: [_ w430 w441 _ w449 _] -> w419
      tunnel: [w429 w431 w439 w442 w448 w457] -> w420
      event Timeout {
        n157 = event-data() -> ()  [unwired: 1 in, 1 out]
      }
      event Panel Close? {
        w433 = TRUE  # Priority Message
        n158 = event-data() -> ()  [unwired: 1 in, 1 out]
        n159 = call-poly "Enqueue Message.vi"("Priority Message? (F)"=w433, "Message"="Confirm Quit", "Message Queue"=w432) -> ("error out"=w430:errorcluster, "dup Message Queue"=w431:refnum<queue>)  [unwired: 7 in]
        n160 = event-data("Discard?"=TRUE) -> ()  [unwired: 1 in, 1 out]
      }
      event "Exit": Value Change {
        w437 = TRUE  # Priority Message
        # "The UI Message Loop handles sending the Exit message to other loops."
        n161 = event-data() -> ()  [unwired: 1 in, 1 out]
        n162 = call-poly "Enqueue Message.vi"("Priority Message? (F)"=w437, "Message"="Exit", "Message Queue"=w436) -> ("error out"=w441:errorcluster, "dup Message Queue"=w439:refnum<queue>)  [unwired: 7 in]
      }
      event User Event {
        # "The Message Handling Loop processed an \"Exit\" message, which fired this event to stop the Event Handling Loop."
        n163 = event-data() -> ()  [unwired: 1 in, 1 out]
        n164 = local write "Status"("Exit" ("Exit String")) -> ()
      }
      event "Settings Button": Mouse Down {
        # "Allow debugging during run with a ctrl click"
        n165 = event-data() -> ("PlatMods"=w446:T9)  [unwired: 1 in]
        n166 = Unbundle By Name(w446) -> ("Ctrl"=w445:bool)
        n167 = case shown="False" w445 {
          tunnel: [w453 w454] -> w449
          tunnel: [w452 w455] -> w448
          tunnel: w447 -> [w451 w455]
          frame False {
            n168 = call-poly "Enqueue Message.vi"("Message"="Launch Settings Dialog", "Message Queue"=w451) -> ("error out"=w453:errorcluster, "dup Message Queue"=w452:refnum<queue>)  [unwired: 8 in]
          }
          frame True {
            n169 = property class="VI"("BDWin.Open"=TRUE ("Block Diagram Window:Open")) -> (error out=w454:errorcluster)  [unwired: 2 in, 1 out]
          }
        }
      }
      event Key Down {
        n170 = event-data() -> ("ScanCode"=→"ScanCode":i16)  [unwired: 1 in]
      }
    }
    n171 = call "Error Handler - Event Handling Loop.vi"("error in (no error)"=w419, "Message Queue"=w420) -> ("dup error in"=w418:errorcluster)  [unwired: 8 in, 1 out]
  }
  n172 = call "Main Loop.vi"("error in (no error)"=w7, "Chart Notifier"=w21, "Message Queues"=w6) -> ("error out"=w22:errorcluster)  [unwired: 8 in]
  n173 = Unregister For Events(event registration refnum=w29, error in=w34) -> (error out=w30:errorcluster)
  n174 = Close Reference(reference=w20) -> ()  [unwired: 1 in, 1 out]
  n175 = Merge Errors(w30, w35, w7, w22) -> (w33:errorcluster)
  n176 = call "Destroy User Event - Stop.vi"("error in (no error)"=w33, "User Event - Stop"=w31) -> ("error out"=w3:errorcluster)  [unwired: 9 in]
  n177 = flat-sequence {
    tunnel: w3 -> [_]
    frame #0 {
      n178 = invoke class="VI" method="FP.Close"() -> ()  [unwired: 3 in, 3 out]
    }
  }
